vi "kindofbinary.vi"(8 "error in (no error)":errorcluster, 11 "selected \"*.dat\" path":path) -> (0 "error out":errorcluster, 1 "what kind of binary":i32, 4 "output path":path)   [LabVIEW 2014]
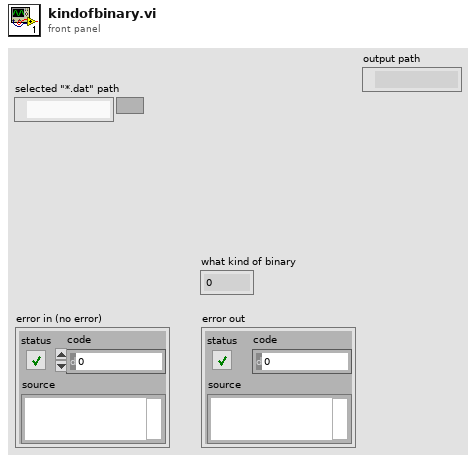
[diagram p1: front panel]
types:
  T1 = enum16{"open", "replace", "create", "open or create", "replace or create", "replace or create with confirmation"}
  T2 = enum16{"deny read/write", "deny write-only", "deny none"}
  T3 = enum16{"big-endian, network order", "native, host order", "little-endian"}
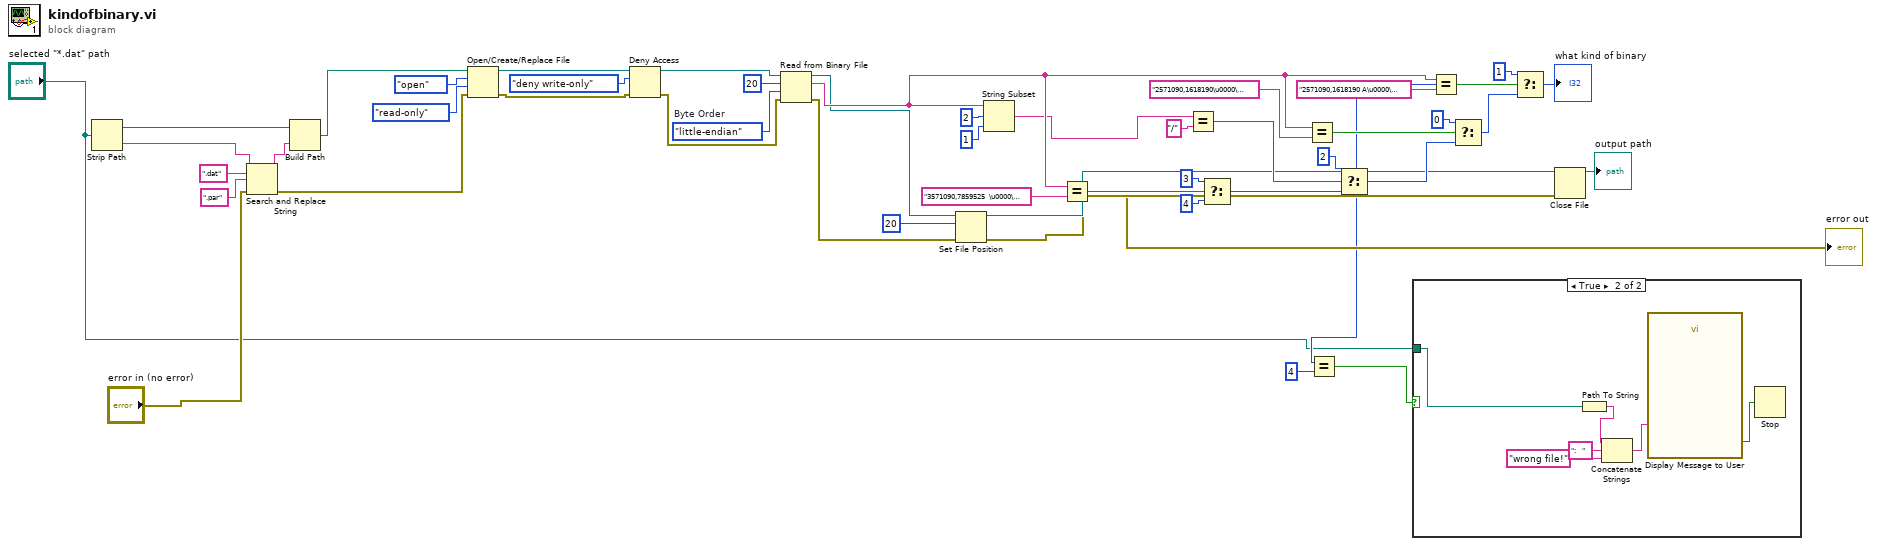
[diagram p0: block diagram]
diagram:
  w18 = T3."little-endian"  # Byte Order
  n1 = Strip Path(path="selected \"*.dat\" path") -> (stripped path=w41:path, name=w42:string)
  n2 = Search and Replace String(input string=w42, search string=".dat", replace string=".par" ("replace string (\"\")"), error in="error in (no error)") -> (result string=w45:string, error out=w48:errorcluster)  [unwired: 4 in, 2 out]
  n3 = Build Path(base path=w41, name or relative path=w45) -> (appended path=w46:path)
  n4 = Open/Create/Replace File(file path (use dialog)=w46, error in=w48, operation (0:open)=T1."open", access (0:read/write)=enum16{"read/write", "read-only", "write-only"}."read-only") -> (refnum out=w16:refnum<file>, error out=w17:errorcluster)  [unwired: 2 in, 1 out]
  n5 = Deny Access(4:w17, 6:T2."deny write-only" ("deny mode (0:deny read/write)"), 7:w16) -> (0:w12:errorcluster, 3:w13:refnum<file>)
  n6 = Read from Binary File(8:w12, 9:w18, 10:20 ("count (1)"), 11:w13) -> (0:w9:errorcluster, 2:w36:string, 3:w11:refnum<file>)  [unwired: 2 in, 1 out]
  n7 = Set File Position(offset (in bytes) (0)=i64 20, refnum=w11, error in=w9) -> (refnum out=w8:refnum<file>, error out=w7:errorcluster)  [unwired: 1 in]
  n8 = String Subset(string=w36, offset (0)=2, length (rest)=1 ("length (rest)")) -> (substring=w30:string)
  n9 = Equal?(x=w36, y="3571090,7859525  \u0000\u0000\u0000" ("String 2")) -> (x = y?=w37:bool)
  n10 = Equal?(x=w30, y="/") -> (x = y?=w32:bool)
  n11 = Select(t=3 ("f"), s=w37, f=4) -> (s? t:f=w40:i32)
  n12 = Equal?(x=w36, y="2571090,1618190\u0000\u0000\u0000\u0000\u0000" ("String 2")) -> (x = y?=w25:bool)
  n13 = Select(t=2 ("offset (0)"), s=w32, f=w40) -> (s? t:f=w34:i32)
  n14 = Equal?(x=w36, y="2571090,1618190 A\u0000\u0000\u0000" ("String 2")) -> (x = y?=w23:bool)
  n15 = Select(t=i16 0, s=w25, f=w34) -> (s? t:f=w27:i32)
  n16 = Select(t=i16 1, s=w23, f=w27) -> (s? t:f=w4:i32)
  "what kind of binary" <- w4
  n17 = Equal?(x=w4, y=4) -> (x = y?=w2:bool)
  n18 = case shown="True" w2 {
    tunnel: "selected \"*.dat\" path" -> [_ w50]
    frame False {
    }
    frame True {
      n19 = Path To String(path=w50) -> (string=w54:string)
      n20 = Concatenate Strings(w54, ":   " ("string"), "wrong file!" ("string")) -> (w51:string)
      n21 = call "Display Message to User"("Message"=w51) -> ("OK"=w49:bool)  [unwired: 9 in, 1 out]
      n22 = Stop(stop? (T)=w49) -> ()
    }
  }
  n23 = Close File(refnum=w8, error in=w7) -> (path=→"output path":path, error out=→"error out":errorcluster)
